vi "set_ThreadPoolReference.vi"(0 "Host_Reference":refnum<class "HGF_Reference.lvclass">, 2 "timeout in ms (-1)":i32=-1, 3 "Threadpool Reference":refnum<class "HGF_Reference.lvclass">, 5 "error in (no error)":errorcluster) -> (14 "dup Host_Reference":refnum<class "HGF_Reference.lvclass">, 19 "error out":errorcluster)   [LabVIEW 2009, in "MoAgSy.lvlib" / "MoAgSy_Host.lvclass"]
doc: "<B>public</B> VI sets threadpool reference for referenced Host.\n\nF.Berck@gsi.de\nGSI Darmstadt 2009"
uses:
  MoAgSy_Host.lvclass
  HGF_BaseClasses/HGF_Reference/HGF_Reference.lvclass
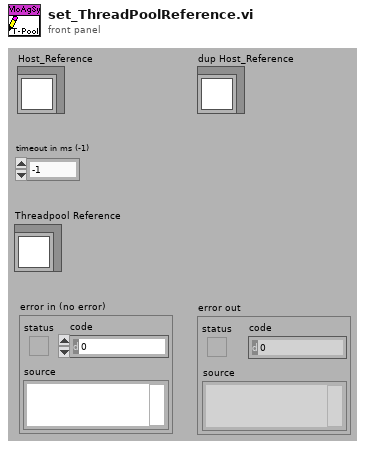
[diagram p1: front panel]
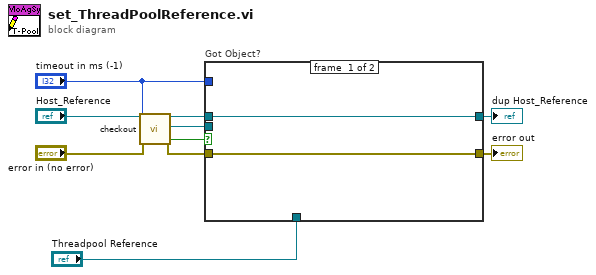
[diagram p0: block diagram]
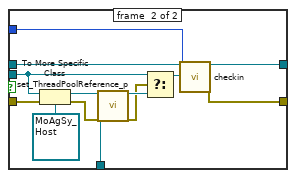
[diagram p2: hidden frame]
diagram:
  n1 = call "checkout.vi"("HGF_Reference"="Host_Reference", "timeout in ms (-1)"="timeout in ms (-1)", "error in (no error)"="error in (no error)") -> ("dup HGF_Reference"=w7:refnum<class "HGF_Reference.lvclass">, "Object"=w9:refnum<class>, "got object?"=w8:bool, "error out"=w10:errorcluster)  [unwired: 13 out]
  n2 = case "Got Object?" shown="True" w8 {
    tunnel: w9 -> [_ w19]
    tunnel: w7 -> [w12 w24]
    tunnel: [w12 w23] -> w3
    tunnel: "timeout in ms (-1)" -> [_ w22]
    tunnel: [w11 w21] -> w4
    tunnel: w10 -> [w11 w20]
    tunnel: "Threadpool Reference" -> [_ w13]
    frame #0 {
    }
    frame #1 {
      n3 = To More Specific Class(target class=refnum<class "MoAgSy_Host.lvclass"> refnum ("MoAgSy.lvlib:MoAgSy_Host.lvclass"), reference=w19, error in=w20) -> (specific class reference=w17:refnum<class "MoAgSy_Host.lvclass">, error out=w14:errorcluster)
      n4 = call "set_ThreadPoolReference_p.vi"("MoAgSy_Host"=w17, "ThreadPool_Reference"=w13, "error in (no error)"=w14) -> ("dup MoAgSy_Host"=w16:refnum<class "MoAgSy_Host.lvclass">, "error out"=w15:errorcluster)  [unwired: 15 out]
      n5 = Select(t=w19, s=w15, f=w16) -> (s? t:f=w18:refnum<class>)
      n6 = call "checkin.vi"("HGF_Reference"=w24, "Object"=w18, "timeout /ms (-1)"=w22) -> ("dup HGF_Reference"=w23:refnum<class "HGF_Reference.lvclass">, "error out"=w21:errorcluster)  [unwired: 1 in, 14 out]
    }
  }
  "dup Host_Reference" <- w3
  "error out" <- w4
